vi "PH_Beckhoff-16BB.START PSDB THREAD.vi"(0 "VI in":refnum<vi>, 5 "error in (no error)":errorcluster) -> (14 "VI out":refnum<vi>, 19 "error out":errorcluster)   [LabVIEW 2014, in "PH_Beckhoff-16BB.lvlib"]
uses:
  PH_Beckhoff-16BB.lvlib
  CS_Core/CSSystem/CSSystemLib/CSSystemLib.lvlib
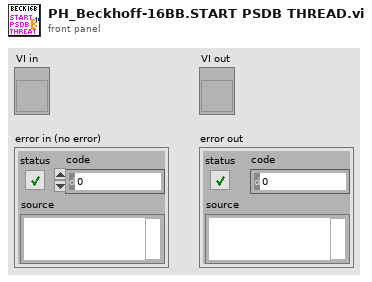
[diagram p1: front panel]
types:
  T1 = typedef "PH_Beckhoff-16BB.lvlib/PH_Beckhoff-16BB.i attribute.ctl" = cluster{"PA Chiller":cluster{"PSDB":cluster{"Status Service ID":i32, "Instance ID":i32, "Data Status":T2, "Ref Status":refnum<vi>, "Error Code":i32}, "Status":cluster{"GUI Ref":refnum<vi>, "Status Service ID":i32, "Status":T3}, "DIs":cluster{"Flow Control":cluster{"GUI Ref":refnum<vi>, "# in Data":i32}, "High-Temp":cluster{"GUI Ref":refnum<vi>, "# in Data":i32}, "Conductivity":cluster{"GUI Ref":refnum<vi>, "# in Data":i32}, "Niveau":cluster{"GUI Ref":refnum<vi>, "# in Data":i32}}, "PSDB Thread":cluster{"Ref":refnum<vi>, "Q-Ref":refnum<queue>}}, "PSDB":cluster{"Shot #":i32, "Subsystem":T4}, "Racktype":string, "PSDB Credentials":T5}
  T2 = typedef "PH_PSDBWriter.lvlib/PH_PSDBWriter.Data Status.ctl" = i16
  T3 = typedef "PH_StatusHandler.lvlib/PH_StatusHandler.Status.ctl" = i16
  T4 = typedef "PH_PSDBWriter.lvlib/PH_PSDBWriter.PHELIX-Subsystems.ctl" = i32
  T5 = typedef "PH_Common.lvlib/PH_Connection.PSDB Credentials.ctl" = cluster{"PW":string, "ID":string, "DS":string}
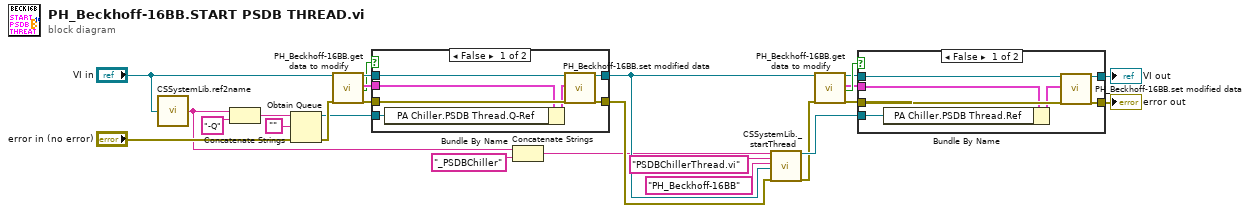
[diagram p0: block diagram]
diagram:
  n1 = call "CSSystemLib.ref2name.vi"("obj refnum"="VI in") -> ("name"=w3:string)
  n2 = Concatenate Strings(w3, "-Q" ("string")) -> (w9:string)
  n3 = Obtain Queue(name (unnamed)=w9, element data type="", error in (no error)="error in (no error)") -> (queue out=w24:refnum<queue>, error out=w26:errorcluster)  [unwired: 2 in, 1 out]
  n4 = call "PH_Beckhoff-16BB.get data to modify.vi"("i ref in"="VI in", "error in (no error)"=w26) -> ("i ref out"=w21:refnum<vi>, "i attribute"=w19:T1, "timed out"=w18:bool, "error out"=w20:errorcluster)  [unwired: 14 in]
  n5 = case shown="False" w18 {
    tunnel: w21 -> [w33 w35]
    tunnel: [w32 w35] -> w23
    tunnel: w20 -> [w31 w34]
    tunnel: [w30 w34] -> w5
    tunnel: w19 -> [w29 _]
    tunnel: w24 -> [w27 _]
    frame False {
      n6 = Bundle By Name(cluster=w29, "PA Chiller.PSDB Thread.Q-Ref"=w27) -> (w28:T1)
      n7 = call "PH_Beckhoff-16BB.set modified data.vi"("i ref in"=w33, "i attribute"=w28, "error in (no error)"=w31) -> ("i ref out"=w32:refnum<vi>, "error out"=w30:errorcluster)  [unwired: 15 in]
    }
    frame True {
    }
  }
  n8 = Concatenate Strings(w3, "_PSDBChiller" ("thread name")) -> (w1:string)
  n9 = call "CSSystemLib._startThread.vi"("thread name"=w1, "template name"="PSDBChillerThread.vi", "Class"="PH_Beckhoff-16BB", "object ref"=w23, "error in (no error)"=w5) -> ("thread ref"=w16:refnum<vi>, "error out"=w13:errorcluster)  [unwired: 12 in, 1 out]
  n10 = call "PH_Beckhoff-16BB.get data to modify.vi"("i ref in"=w23, "error in (no error)"=w13) -> ("i ref out"=w10:refnum<vi>, "i attribute"=w15:T1, "timed out"=w17:bool, "error out"=w12:errorcluster)  [unwired: 14 in]
  n11 = case shown="False" w17 {
    tunnel: w10 -> [w42 w44]
    tunnel: [w41 w44] -> w11
    tunnel: w12 -> [w40 w43]
    tunnel: [w39 w43] -> w14
    tunnel: w15 -> [w38 _]
    tunnel: w16 -> [w36 _]
    frame False {
      n12 = Bundle By Name(cluster=w38, "PA Chiller.PSDB Thread.Ref"=w36) -> (w37:T1)
      n13 = call "PH_Beckhoff-16BB.set modified data.vi"("i ref in"=w42, "i attribute"=w37, "error in (no error)"=w40) -> ("i ref out"=w41:refnum<vi>, "error out"=w39:errorcluster)  [unwired: 15 in]
    }
    frame True {
    }
  }
  "error out" <- w14
  "VI out" <- w11
